vi "fmTest_MQTT_Simple_Connect_and_Publish.vi"() -> ()   [LabVIEW 2018]
doc: "A simple client example that connects to a broker server and publishes messages to a topic.\n\n© 2015 - daq.io, LLC - Peter Adelhardt"
uses:
  source/support/mqtt/Controls/QoS.ctl
  source/support/mqtt/Controls/Retain_Flag.ctl
  source/support/mqtt/Controls/DUP_Flag.ctl
  source/support/mqtt/Controls/Connection_Return_Codes.ctl
  source/support/mqtt/Controls/Connect_Flags.ctl
  source/support/mqtt/MQTT_Functions.lvlib
panel:
  out "message count":i32=16
  in  "rate":u32=1000
  out "Message published":string="LabVIEW says it's 17:46:03"
  in  "Stop Publishing":bool
  out "Message ID (acknowledged)":u16=10
  out "Acknowledged":bool
  in  "Message ID":u16=20
  in  "MQTT Broker":cluster{"address (IP)":string, "port":u16}={"address (IP)"="192.168.52.151", "port"=1883}
  in  "Message to be published":string="LabVIEW says it's "
  out "Connection Status":T1
  out "error out":errorcluster
  in  "Client ID":string="LVSubscribeClient2"
  in  "error in (no error)":errorcluster
  in  "Topic":string="home/garden/fountain"
  in  "Publish Meta":cluster{"QoS":T2, "Retain":T3, "DUP":T4}
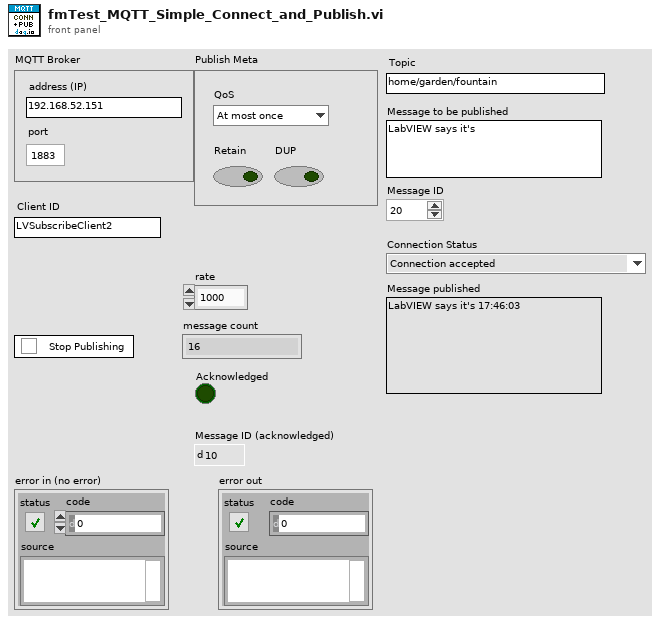
[diagram p1: front panel]
types:
  T1 = typedef "MQTT_Functions.lvlib/Connection_Return_Codes.ctl" = enum16{"Connection accepted", "Connection refused: unacceptable protocol version", "Connection refused: identifier rejected", "Connection refused: Server unavailable", "Connection refused: bad user name or password", "Connection refused: not authorized"}
  T2 = typedef "MQTT_Functions.lvlib/QoS.ctl" = enum8{"At most once", "At least once", "Exactly once", "Reserved"}
  T3 = typedef "MQTT_Functions.lvlib/Retain_Flag.ctl" = bool
  T4 = typedef "MQTT_Functions.lvlib/DUP_Flag.ctl" = bool
  T5 = typedef "MQTT_Functions.lvlib/Connect_Flags.ctl" = cluster{"user name":bool, "password":bool, "will retain":bool, "will flag":bool, "clean session":bool, "reserved":bool, "will QoS":T2}
  T6 = cluster{"QoS":T2, "DUP":T4, "Retain":T3, "Keep Alive (sec)":u16}
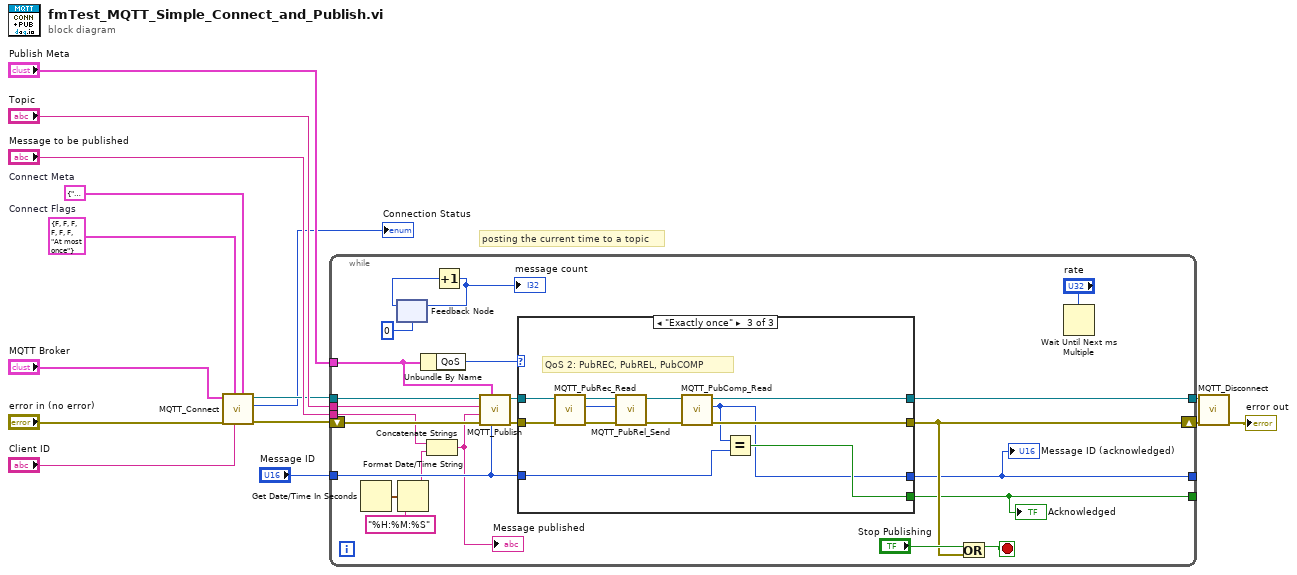
[diagram p0: block diagram]
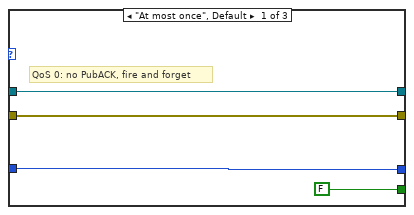
[diagram p2: hidden frame]
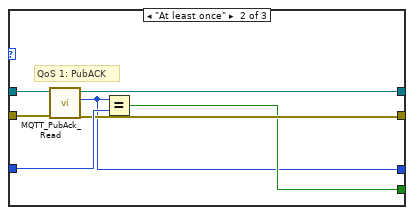
[diagram p3: hidden frame]
diagram:
  w13 = T5 {"user name"=FALSE, "password"=FALSE, "will retain"=FALSE, "will flag"=FALSE, "clean session"=FALSE, "reserved"=FALSE, "will QoS"=enum."At most once"}  # Connect Flags
  w10 = T6 {"QoS"=enum."At most once", "DUP"=FALSE, "Retain"=FALSE, "Keep Alive (sec)"=60}  # Connect Meta
  # "posting the current time to a topic"
  n1 = call "MQTT_Connect.vi"("Connect Meta"=w10, "Client ID"="Client ID", "Connect Flags"=w13, "error in (no error)"="error in (no error)", "MQTT Broker"="MQTT Broker") -> ("error out"=w1:errorcluster, "Connection Status"=→"Connection Status":T1, "connection ID out"=w3:refnum<k5>)  [unwired: 4 in]
  n2 = while {
    tunnel: "Topic" -> [w38]
    tunnel: "Message to be published" -> [w28]
    tunnel: w3 -> [w37]
    tunnel: "Publish Meta" -> [w35]
    tunnel: [w31] -> w6
    tunnel: "Message ID" -> [w30]
    tunnel: [w20] -> _
    tunnel: [w19] -> _
    shift-right: [w22] -> w7
    shift-left: w1 -> [w36]
    stop <- w23 stop-if-true
    n3 = Get Date/Time In Seconds() -> (seconds since 1Jan1904=w27:timestamp)
    n4 = feedback #1(0) -> (w17:i32)
    n5 = Format Date/Time String(time format string (%c)="%H:%M:%S", seconds (now)=w27) -> (date/time string=w25:string)  [unwired: 1 in]
    n6 = Unbundle By Name(w35) -> ("QoS"=w34:T2)
    n7 = Concatenate Strings(w28, w25) -> (w24:string)
    "Message published" <- w24
    n8 = Increment(x=w17) -> (x+1=w16:i32)
    "message count" <- w16
    n9 = feedback-in #1(w16) -> ()
    n10 = call "MQTT_Publish.vi"("Message ID"=w30, "Publish Meta"=w35, "error in (no error)"=w36, "Message to be published"=w24, "Topic"=w38, "connection ID"=w37) -> ("error out"=w33:errorcluster, "connection ID out"=w32:refnum<k5>)  [unwired: 4 in]
    n11 = case shown="\"Exactly once\"" w34 {
      tunnel: w33 -> [w41 w48 w60]
      tunnel: w32 -> [w42 w49 w61]
      tunnel: [w41 w46 w53] -> w22
      tunnel: [w42 w45 w54] -> w31
      tunnel: w30 -> [w39 w47 w59]
      tunnel: [FALSE w44 w55] -> w20
      tunnel: [w39 w43 w52] -> w19
      frame "At most once", Default {
        # "QoS 0: no PubACK, fire and forget"
      }
      frame "At least once" {
        # "QoS 1: PubACK"
        n12 = call "MQTT_PubAck_Read.vi"("error in (no error)"=w48, "connection ID"=w49) -> ("error out"=w46:errorcluster, "Message ID"=w43:u16, "connection ID out"=w45:refnum<k5>)  [unwired: 7 in]
        n13 = Equal?(x=w43, y=w47) -> (x = y?=w44:bool)
      }
      frame "Exactly once" {
        # "QoS 2: PubREC, PubREL, PubCOMP"
        n14 = call "MQTT_PubRec_Read.vi"("error in (no error)"=w60, "connection ID"=w61) -> ("error out"=w58:errorcluster, "Message ID"=w56:u16, "connection ID out"=w57:refnum<k5>)  [unwired: 7 in]
        n15 = call "MQTT_PubRel_Send.vi"("error in (no error)"=w58, "Message ID"=w56, "connection ID"=w57) -> ("error out"=w50:errorcluster, "connection ID out"=w51:refnum<k5>)  [unwired: 6 in, 1 out]
        n16 = call "MQTT_PubComp_Read.vi"("error in (no error)"=w50, "connection ID"=w51) -> ("error out"=w53:errorcluster, "Message ID"=w52:u16, "connection ID out"=w54:refnum<k5>)  [unwired: 7 in]
        n17 = Equal?(x=w52, y=w59) -> (x = y?=w55:bool)
      }
    }
    "Message ID (acknowledged)" <- w19
    "Acknowledged" <- w20
    n18 = Or(x="Stop Publishing", y=w22) -> (x .or. y?=w23:bool)
    n19 = Wait Until Next ms Multiple(millisecond multiple="rate") -> ()  [unwired: 1 out]
  }
  n20 = call "MQTT_Disconnect.vi"("error in (no error)"=w7, "connection ID"=w6) -> ("error out"=→"error out":errorcluster)  [unwired: 9 in]
